vi "Start Call (Exe Name).vi"(6 "Event References":T1, 7 "Configuration":refnum<class "configuration.lvclass">, 8 "error in":errorcluster, 9 "Working Directory (default <Not A Path> - System Default)":path=path "" caption="Working Directory", 10 "Arguments":string, 11 "Executable Name":string) -> (0 "error out":errorcluster, 3 "New ASE Handle":refnum<class "ase.lvclass">)   [LabVIEW 2020, in "serenial.io-ase.lvlib" / "ase.lvclass"]
doc: "<B>Start an Asynchronous System Executable Call</B>\n\nThe name of an executable should be available in this process's PATH variable. The full path of the executable called will be provided by the \"Did Launch\" User Event.\n\nThe User Events References to generate the \"Did Launch\", \"Standard Output\", \"Standard Error\" and \"Did Exit\" events can be supplied or omitted as required. <B>Ensure that the event registration process for any User Events passed to this VI has already been undertaken</B>.\n\nArguments that are to be passed to the executable are specified in an array. Ensure that each argument specifier or value is in a different array element. E.g. to call the ping executable with the arguments \"-n 10 localhost\" use the element values [ -n, 10, localhost].\n\nThe configuration class allows for override of certain behaviours such as the regular expression used to match the breaks in the Standard Out and Standard Error to be specified.\n\nThis VI generates the following errors:\n-4601: Poorly formatted/incorrect Regular Expression supplied.\n-5691000: Internal Library Error. <Check Error Message for more details>\n-5691301: Unable to launch the executable. <Check Error Message for more details>\n-5691305: Executable name/path parameter cannot be an empty value."
uses:
  ase.lvclass
  Event References.ctl
  Standard Output.ctl
  Standard Error.ctl
  Did Exit.ctl
  configuration/configuration.lvclass
  ase.lvclass/ase.ctl
  Error Internal Library Implementation Error.vi
  <vilib>/dlg_ctls.llb/Space Constant.vi
  <vilib>/Utility/error.llb/Error Cluster From Error Code.vi
  serenial.io-ase.32.dll
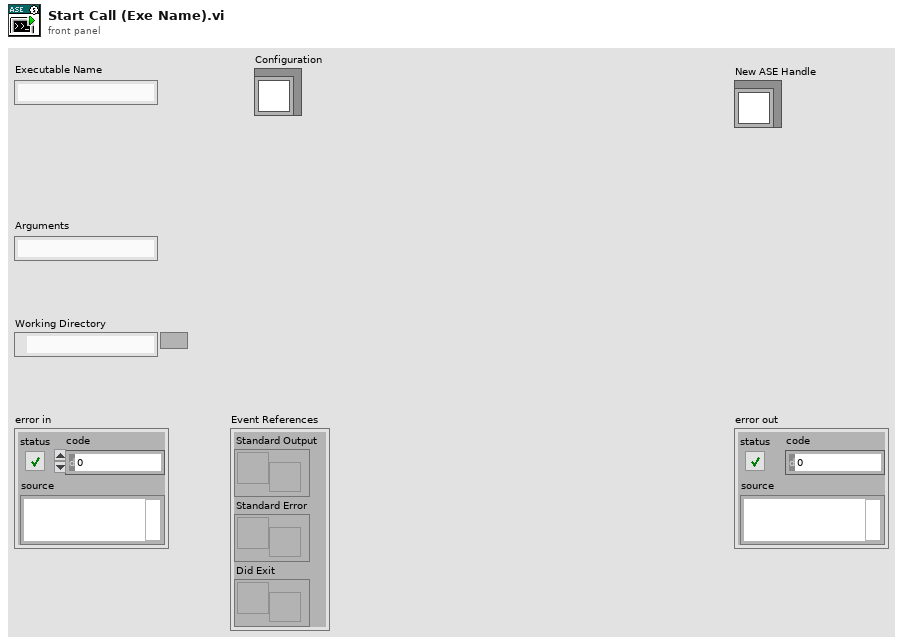
[diagram p1: front panel]
types:
  T1 = typedef "serenial.io-ase.lvlib/ase.lvclass/Event References.ctl" = cluster{"Standard Output":refnum<user-event>, "Standard Error":refnum<user-event>, "Did Exit":refnum<user-event>}
  T2 = cluster{"Stream Split Character Match RegExp Std Out":string, "Stream Split Character Match RegExp Std Err":string}
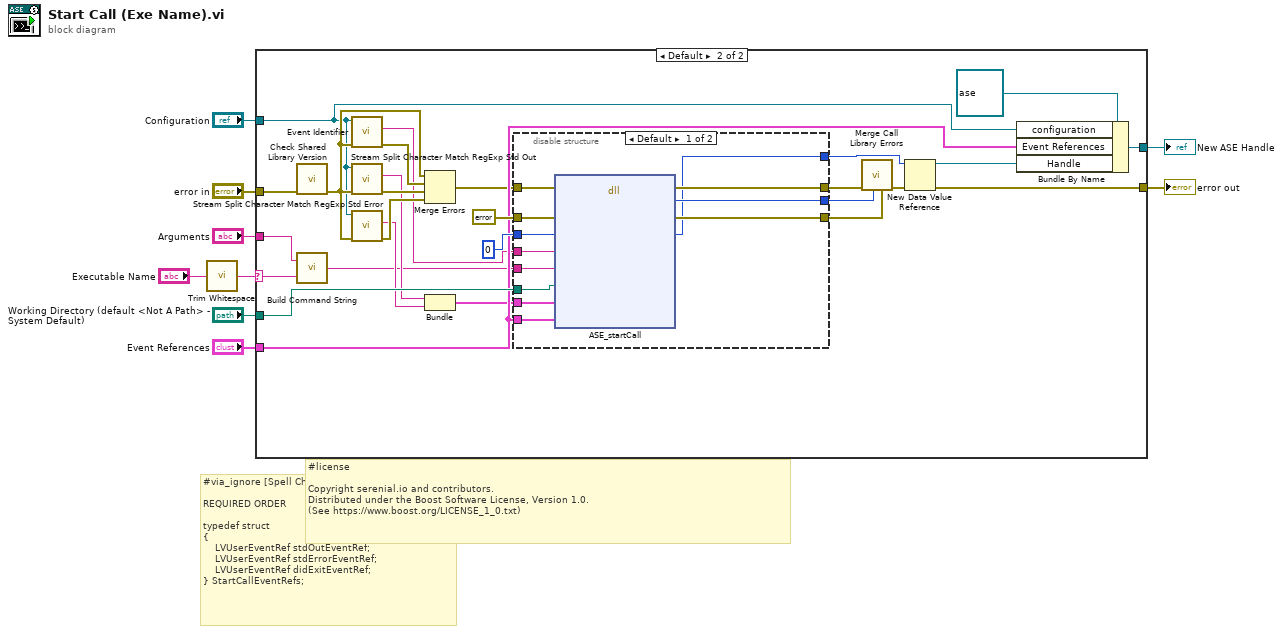
[diagram p0: block diagram]
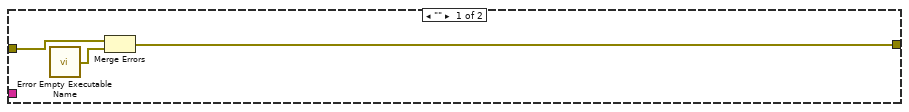
[diagram p2: hidden frame]
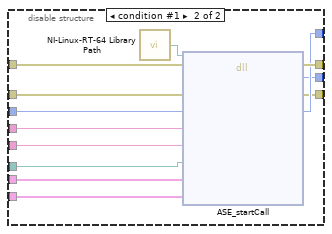
[diagram p3: hidden frame]
diagram:
  # "#license\n\nCopyright serenial.io and contributors.\nDistributed under the Boost Software License, Version 1.0.\n(See https://www.boost.org/LICENSE_1_0.txt)"
  # "#via_ignore [Spell Check]\n\nREQUIRED ORDER\n\ntypedef struct\n{\n    LVUserEventRef stdOutEventRef;\n    LVUserEventRef stdErrorEventRef;\n    LVUserEventRef didExitEventRef;\n} StartCallEventRefs;"
  n1 = call "Trim Whitespace.vi"("Input"="Executable Name") -> ("Output"=w2:string)
  n2 = case shown="Default" w2 {
    selector: w2 -> [_ w15]
    tunnel: "error in" -> [w12 w39]
    tunnel: "Working Directory (default <Not A Path> - System Default)" -> [_ w32]
    tunnel: [_ w36] -> w7
    tunnel: "Event References" -> [_ w31]
    tunnel: [w11 w35] -> w5
    tunnel: "Configuration" -> [_ w18]
    tunnel: "Arguments" -> [_ w14]
    frame "" {
      n3 = call "Error Empty Executable Name.vi"() -> ("Invalid Executable Name"=w10:errorcluster)
      n4 = Merge Errors(w12, w10) -> (w11:errorcluster)
    }
    frame Default {
      n5 = call "Check Shared Library Version.vi"("error in"=w39) -> ("error out"=w25:errorcluster)  [unwired: 10 in]
      n6 = call "Build Command String.vi"("Executable"=w15, "Arguments"=w14) -> ("Command String"=w13:string)
      n7 = call-dynamic "Event Identifier.vi"("error in (no error)"=w25, "configuration in"=w18) -> ("error out"=w24:errorcluster, "Event Identifier"=w20:string)  [unwired: 8 in]
      n8 = call-dynamic "Stream Split Character Match RegExp Std Out.vi"("error in (no error)"=w25, "configuration in"=w18) -> ("error out"=w23:errorcluster, "Stream Split Character Match RegExp Std Out"=w17:string)  [unwired: 8 in]
      n9 = call-dynamic "Stream Split Character Match RegExp Std Error.vi"("error in (no error)"=w25, "configuration in"=w18) -> ("error out"=w22:errorcluster, "Stream Split Character Match RegExp Std Err"=w16:string)  [unwired: 8 in]
      n10 = Merge Errors(w25, w24, w23, w22) -> (w21:errorcluster)
      n11 = Bundle("Stream Split Character Match RegExp Std Out"=w17, "Stream Split Character Match RegExp Std Err"=w16) -> (w26:T2)  [unwired: 1 in]
      n12 = disable-structure "Conditional Disable Structure" shown="Default" {
        disable-tunnel: w21 -> [w51 w64]
        disable-tunnel: errorcluster {"status"=FALSE, "code"=0, "source"=""} ("error in (no error)") -> [w50 w63]
        disable-tunnel: u64 0 ("ASE interface pointer") -> [w49 w62]
        disable-tunnel: w20 -> [w48 w61]
        disable-tunnel: w13 -> [w47 w60]
        disable-tunnel: w32 -> [w46 w59]
        disable-tunnel: w26 -> [w45 w57]
        disable-tunnel: w31 -> [w44 w58]
        disable-tunnel: [w43 w56] -> w30
        disable-tunnel: [w42 w54] -> w29
        disable-tunnel: [w41 w53] -> w28
        disable-tunnel: [w40 w55] -> w27
        frame condition #0 (active) {
          n13 = dll-call lib="C:/serenial/libraries/Asynchronous-System-Executive/LabVIEW/serenial.io-ase/ase/serenial.io-ase.*.*" fn="ASE_startCall"(error in=w51, "Error Out"=w50, "ASE interface pointer"=w49, "ID"=w48, "Command"=w47, "Working Directory"=w46, "Stream Split RegEx"=w45, "Even Refs"=w44) -> (error out=w43:errorcluster, "Error Code"=w42:i32, "Error Out"=w41:errorcluster, "ASE interface pointer"=w40:u64)  [unwired: 7 in, 1 out]
        }
        frame condition #1 {
          n14 = call "NI-Linux-RT-64 Library Path.vi"() -> ("Path"=w52:path)
          n15 = dll-call lib="?" fn="ASE_startCall"(path in=w52, error in=w64, "Error Out"=w63, "ASE interface pointer"=w62, "ID"=w61, "Command"=w60, "Working Directory"=w59, "Stream Split RegEx"=w57, "Even Refs"=w58) -> (error out=w56:errorcluster, "Error Code"=w54:i32, "Error Out"=w53:errorcluster, "ASE interface pointer"=w55:u64)  [unwired: 6 in, 1 out]
        }
      }
      n16 = call "Merge Call Library Errors.vi"("Library Call Returned Error"=w28, "Error Code"=w29, "error in"=w30) -> ("error IO"=w38:errorcluster)  [unwired: 8 in]
      n17 = New Data Value Reference(data value=w27, error in=w38) -> (data value reference=w37:refnum<data-value>, error out=w35:errorcluster)
      n18 = Bundle By Name(cluster=refnum<class "ase.lvclass"> refnum ("serenial.io-ase.lvlib:ase.lvclass"), "configuration"=w18, "Event References"=w31, "Handle"=w37) -> (w36:refnum<class "ase.lvclass">)
    }
  }
  "New ASE Handle" <- w7
  "error out" <- w5
